vi "Read Assertions count.vi"(11 "Method Result In":refnum<class "Method Result.lvclass">) -> (1 "Assertions count string":string, 2 "Assertions count":i32, 3 "Method Result Out":refnum<class "Method Result.lvclass">)   [LabVIEW 2020, in "Method Result.lvclass"]
uses:
  Method Result.lvclass
  Method Result.lvclass/Method Result.ctl
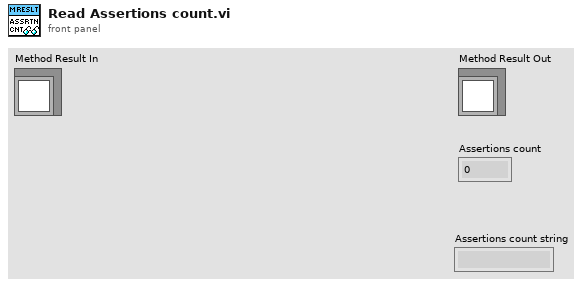
[diagram p1: front panel]
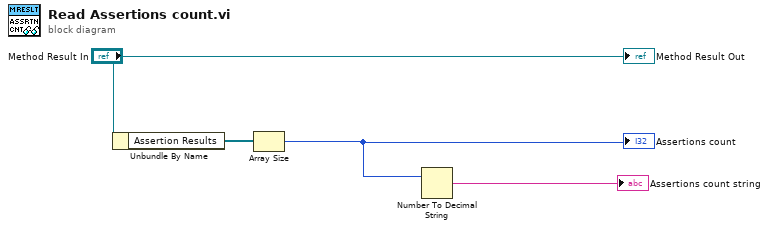
[diagram p0: block diagram]
diagram:
  n1 = Unbundle By Name("Method Result In") -> ("Assertion Results"=w3:refnum<class "Assertion Result.lvclass">[])
  n2 = Array Size(array=w3) -> (size(s)=w1:i32)
  "Assertions count" <- w1
  n3 = Number To Decimal String(number=w1) -> (decimal integer string=→"Assertions count string":string)  [unwired: 1 in]
  "Method Result Out" <- "Method Result In"
